vi "Save File Check For Blanks.vi"(8 "Error In":errorcluster, 9 "Station Index":i32, 10 "Active Stations":bool[](array[boolean]), 11 "Front Panel In":T1 {"Address" format="%x"; "Source" format="%x"}) -> (0 "Error Out":errorcluster, 3 "Blanks (T)":bool)   [LabVIEW 2016]
uses:
  Washer HCC/Washer HCC NEWFI/Type Definitions/HCC Filename Setup.ctl
  Public/Type Definitions/Save File Unit Type.ctl
  Save File.lvlib
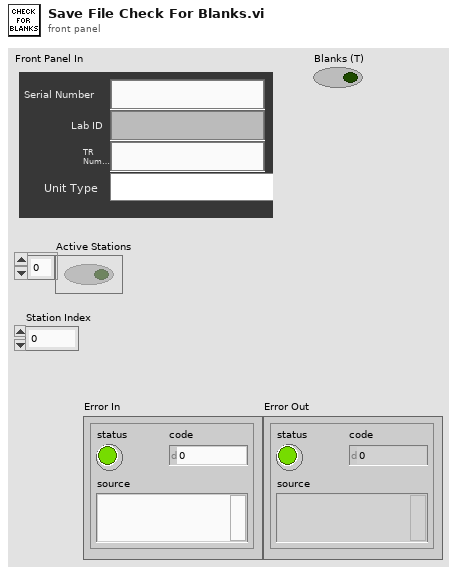
[diagram p1: front panel]
types:
  T1 = typedef "HCC Filename Setup.ctl" = cluster{"Serial Number":string, "Lab ID":string, "TR Number":string, "Unit Type":T2, "Source":u8, "Address":u8}
  T2 = typedef "Save File.lvlib/Save File Unit Type.ctl" = enum32{"", "Viper", "Hawk", "2015"}
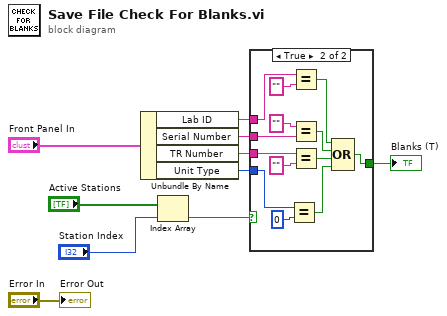
[diagram p0: block diagram]
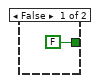
[diagram p2: hidden frame]
diagram:
  n1 = Unbundle By Name("Front Panel In") -> ("Lab ID"=w3:string, "Serial Number"=w2:string, "TR Number"=w4:string, "Unit Type"=w6:T2)
  n2 = Index Array(array="Active Stations", index="Station Index") -> (element=w8:bool)
  n3 = case shown="True" w8 {
    tunnel: w2 -> [_ w24]
    tunnel: w3 -> [_ w23]
    tunnel: w4 -> [_ w22]
    tunnel: [FALSE w21] -> w5
    tunnel: w6 -> [_ w20]
    frame False {
    }
    frame True {
      n4 = Equal?(x=w20, y=u16 0) -> (x = y?=w12:bool)
      n5 = Equal?(x=w23, y="") -> (x = y?=w19:bool)
      n6 = Equal?(x="", y=w24) -> (x = y?=w18:bool)
      n7 = Equal?(x=w22, y="") -> (x = y?=w17:bool)
      n8 = Compound Arithmetic op=OR(w19, w18, w17, w12) -> (w21:bool)
    }
  }
  "Blanks (T)" <- w5
  "Error Out" <- "Error In"
